vi "Tusk.UnwrapMessage.vi"(8 "error in (no error)":errorcluster, 9 "Message":refnum<class "Message.lvclass">, 11 "Tusk in":refnum<class "Tusk.lvclass">) -> (0 "error out":errorcluster, 1 "Data":variant, 2 "Message":string, 3 "Tusk out":refnum<class "Tusk.lvclass">, 4 "Sender":string, 5 "Time Sent":timestamp)   [LabVIEW 2018, in "Application.lvlib" / "Tusk.lvclass"]
uses:
  Tusk.lvclass
  Message Class/Message.lvclass
  Tusk.lvclass/Tusk.ctl
  Message Class/Message.lvclass/Message.ctl
  Keywords Class/Keywords.lvclass
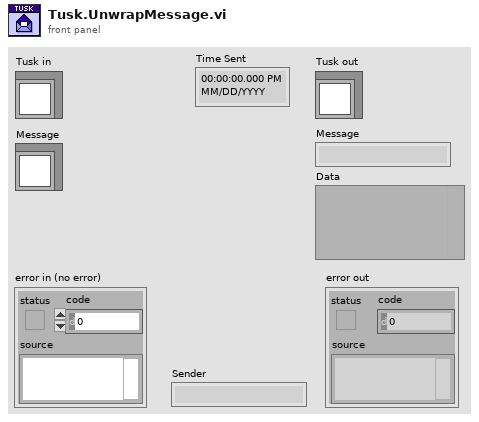
[diagram p1: front panel]
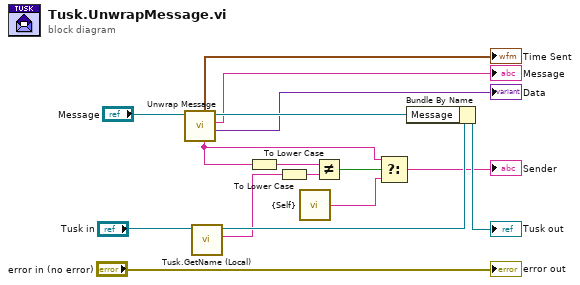
[diagram p0: block diagram]
diagram:
  n1 = call "Unwrap Message.vi"("Message in"="Message") -> ("Data"=→"Data":variant, "Message"=→"Message":string, "Message out"=w13:refnum<class "Message.lvclass">, "Sender"=w3:string, "Time Sent"=→"Time Sent":timestamp)  [unwired: 5 in, 1 out]
  n2 = call "Tusk.GetName (Local).vi"("Tusk in"="Tusk in") -> ("Name(Local)"=w7:string, "Tusk out"=w8:refnum<class "Tusk.lvclass">)  [unwired: 8 in, 1 out]
  n3 = To Lower Case(string=w3) -> (all lower case string=w5:string)
  n4 = To Lower Case(string=w7) -> (all lower case string=w4:string)
  n5 = call "{Self}.vi"() -> ("Word"=w1:string)  [unwired: 6 in]
  n6 = Not Equal?(x=w5, y=w4) -> (x != y?=w6:bool)
  n7 = Select(t=w3, s=w6, f=w1) -> (s? t:f=→"Sender":string)
  n8 = Bundle By Name(cluster=w8, "Message"=w13) -> (→"Tusk out":refnum<class "Tusk.lvclass">)
  "error out" <- "error in (no error)"
